vi "AEcollector.vi"() -> ()   [LabVIEW 2009]
panel:
  out "Ch ctrl":bool[](array[boolean])
  out "Channel count":i32
  out "First trigger signal time":timestamp
  out "Boolean 2":bool
  out "# elements in writing queue":i32
  out "Saving data?":bool
  out "Writing loop":bool
  out "Prefilter loop":bool
  out "Collection loop":bool
  out "stateError":bool
  out "stopCollection":bool
  out "# elements in prefiltering queue":i32
  out "Prefiltering loop":i32
  out "Max event amplitude":dbl(knob) scale=0.0..1.0
  out "Data collection loop":i32
  out "data writing loop":i32
  out "Data stream":dynamicdata(graph)
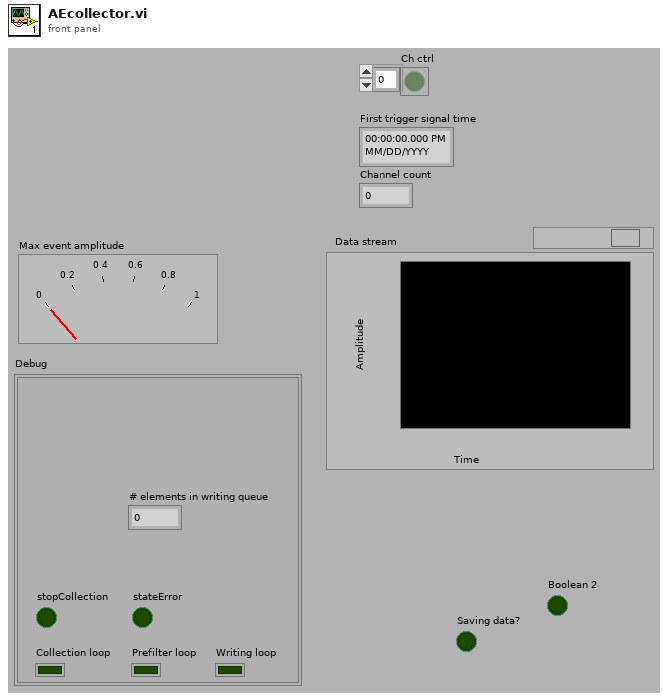
[diagram p1: front panel]
types:
  T1 = enum16{"Read", "Write", "ReadWrite", "BufferedRead", "BufferedReadWrite"}
  T2 = enum16{"open", "replace", "create", "open or create", "replace or create", "replace or create with confirmation"}
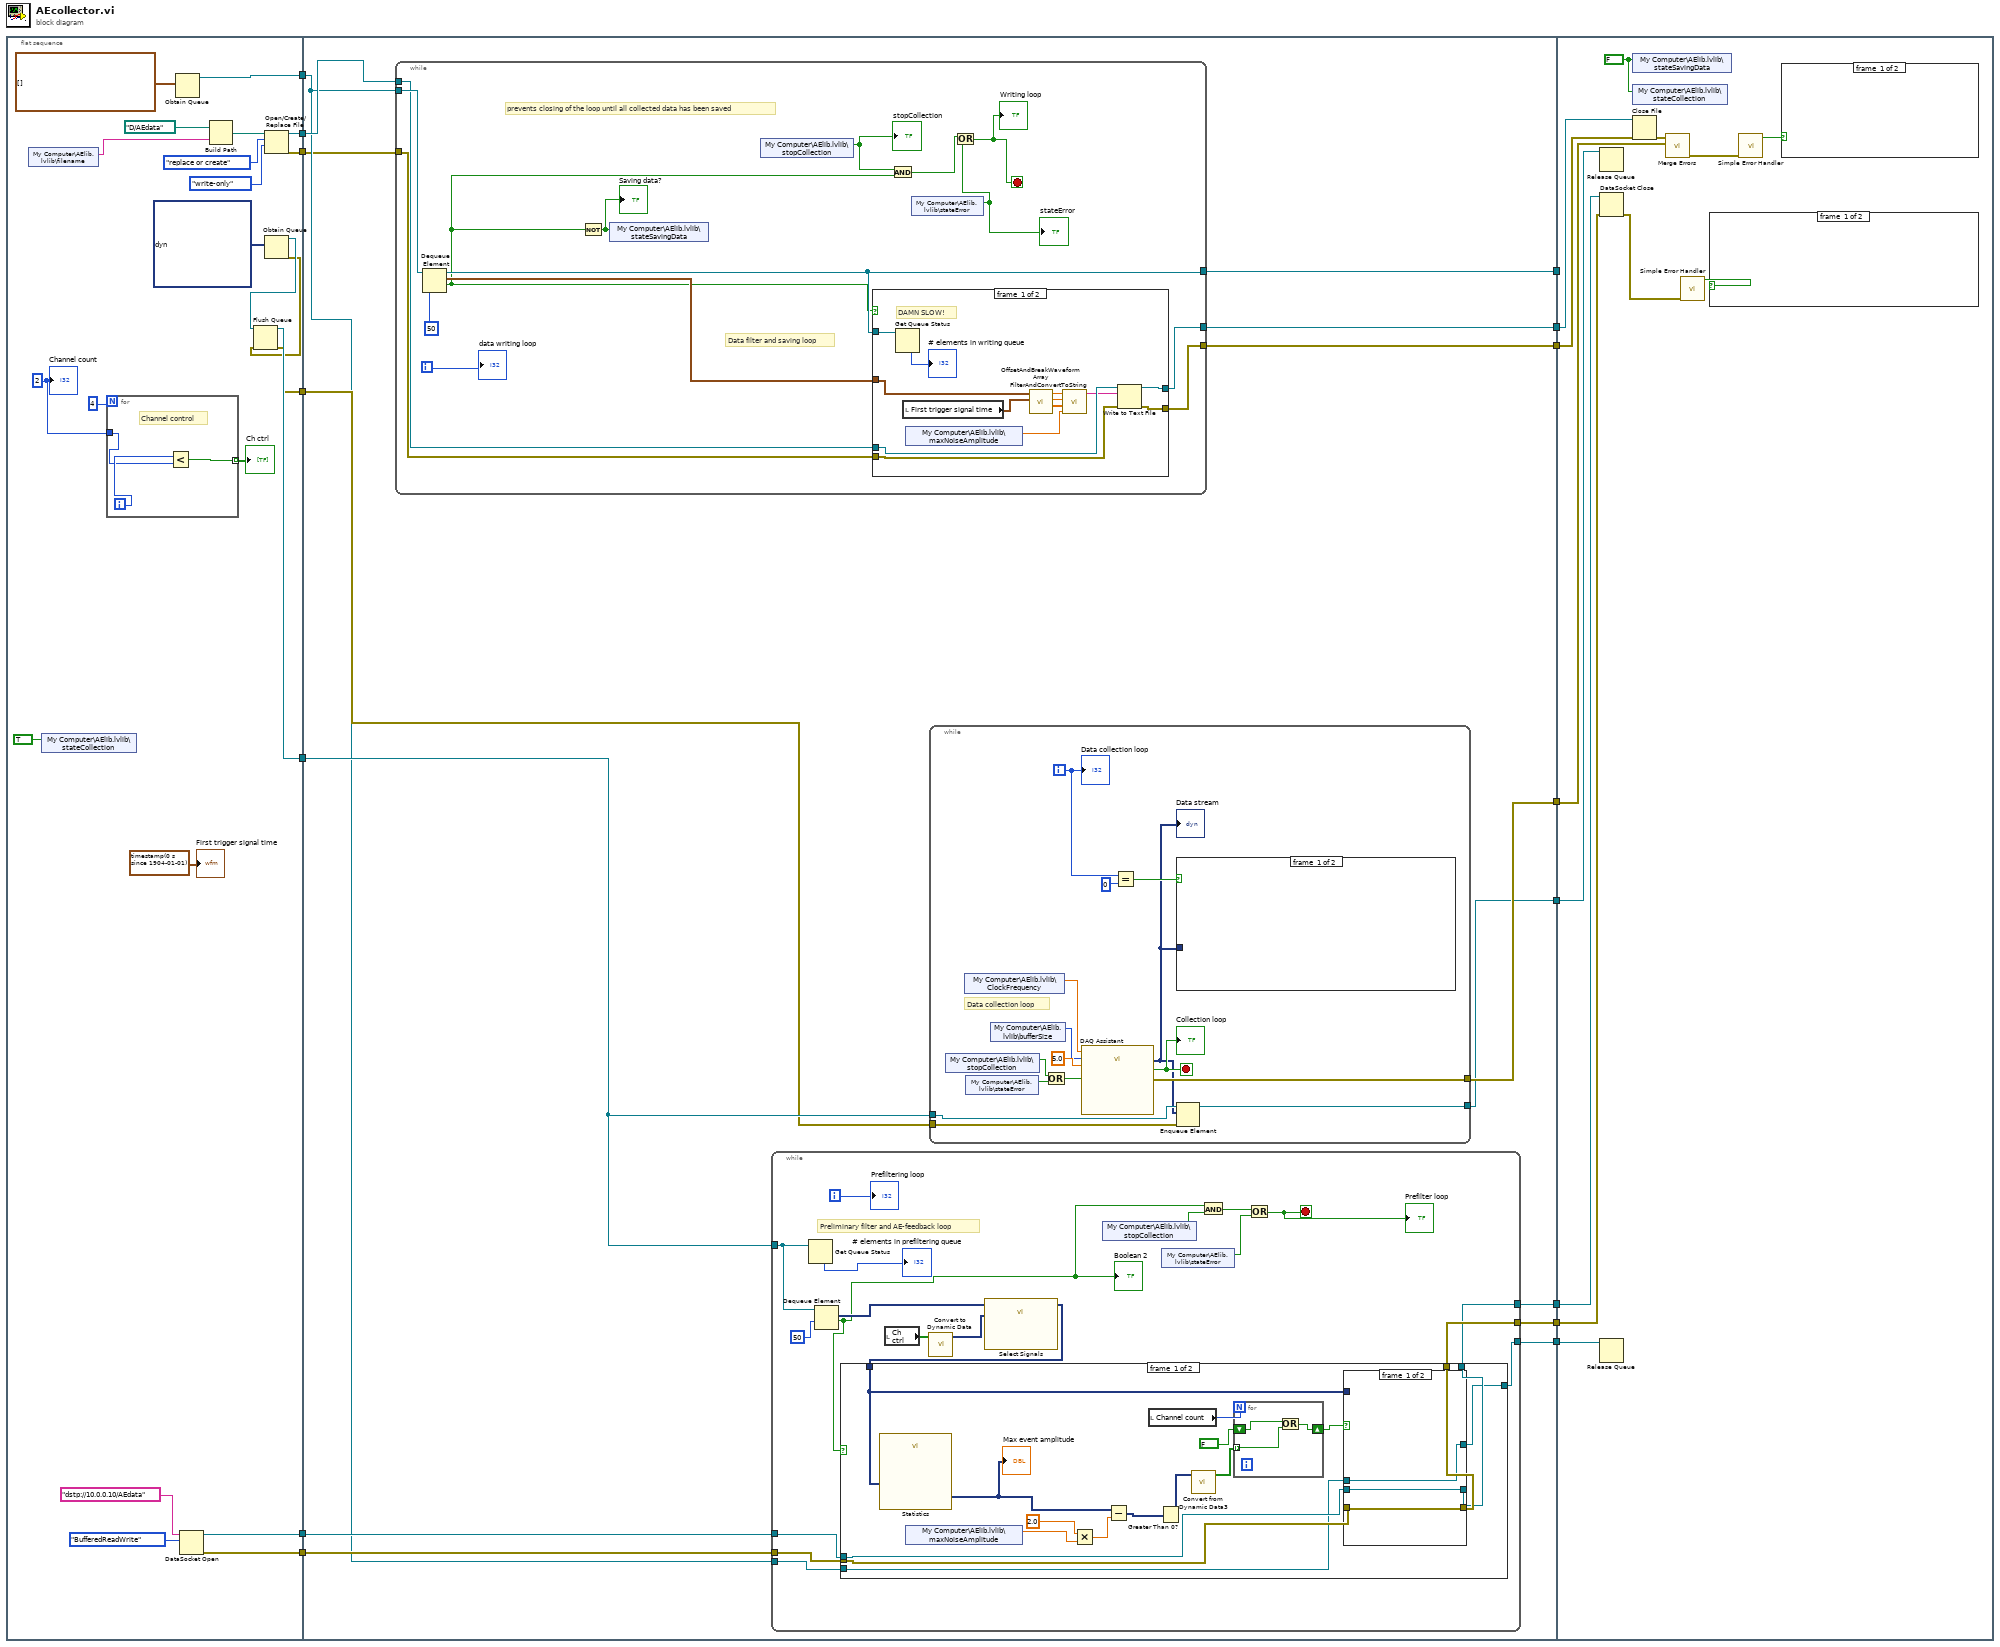
[diagram p0: block diagram]
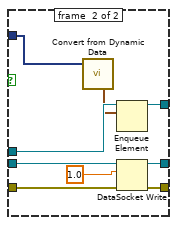
[diagram p2: hidden frame]
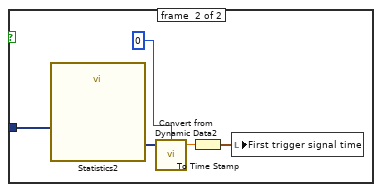
[diagram p5: hidden frame]
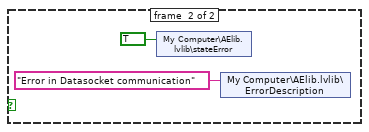
[diagram p6: hidden frame]
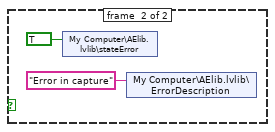
[diagram p7: hidden frame]
diagram:
  n1 = flat-sequence {
    tunnel: [w35] -> w13
    tunnel: [w32] -> w12
    tunnel: [w31] -> w11
    tunnel: [w30] -> w9
    tunnel: [w25] -> w8
    tunnel: [w24] -> w7
    tunnel: [w27] -> w2
    tunnel: [w56] -> w15
    tunnel: [w55] -> w14
    tunnel: w13 -> [w54]
    tunnel: w12 -> [w52]
    tunnel: w11 -> [w53]
    tunnel: [w51] -> w10
    tunnel: w9 -> [w46]
    tunnel: w8 -> [w50]
    tunnel: w7 -> [w49]
    tunnel: [w48] -> w6
    tunnel: [w47] -> w5
    tunnel: [w45] -> w4
    tunnel: [w44] -> w3
    tunnel: w2 -> [w43]
    tunnel: [w42] -> w1
    tunnel: w15 -> [w166]
    tunnel: w14 -> [_]
    tunnel: w10 -> [w172]
    tunnel: w6 -> [w171]
    tunnel: w5 -> [w163]
    tunnel: w4 -> [w170]
    tunnel: w3 -> [w169]
    tunnel: w1 -> [w168]
    frame #0 {
      w19 = 2
      n2 = shared-variable "My Computer\\AElib.lvlib\\filename"() -> (w16:string)  [unwired: 1 in, 1 out]
      n3 = shared-variable "My Computer\\AElib.lvlib\\stateCollection"(TRUE ("stateCollection")) -> ()  [unwired: 1 in, 1 out]
      n4 = for {
        N: 4 -> [_]
        tunnel: w19 -> [w40]
        tunnel: [w39] -> w18 mode=indexing
        i -> [w41]
        # "Channel control"
        n5 = Less?(x=w41, y=w40) -> (x < y?=w39:bool)
      }
      "Ch ctrl" <- w18
      n6 = Obtain Queue(element data type=waveform(dbl)[] []) -> (queue out=w30:refnum<queue>)  [unwired: 4 in, 2 out]
      n7 = DataSocket Open(10:T1."BufferedReadWrite" ("mode"), 11:"dstp://10.0.0.10/AEdata" ("URL")) -> (0:w32:errorcluster, 3:w31:refnum<k13>)  [unwired: 2 in]
      n8 = Build Path(base path=path "D:/AEdata", name or relative path=w16) -> (appended path=w28:path)
      n9 = Open/Create/Replace File(file path (use dialog)=w28, operation (0:open)=T2."replace or create", access (0:read/write)=enum16{"read/write", "read-only", "write-only"}."write-only") -> (refnum out=w35:refnum<file>, error out=w27:errorcluster)  [unwired: 3 in, 1 out]
      n10 = Obtain Queue(element data type=dynamicdata [] ("RMS")) -> (queue out=w26:refnum<queue>, error out=w23:errorcluster)  [unwired: 4 in, 1 out]
      n11 = Flush Queue(queue=w26, error in (no error)=w23) -> (queue out=w25:refnum<queue>, error out=w24:errorcluster)  [unwired: 1 out]
      "First trigger signal time" <- timestamp(0 s since 1904-01-01) ("Time Stamp")
      "Channel count" <- w19
    }
    frame #1 {
      n12 = while {
        tunnel: w54 -> [w115]
        tunnel: w46 -> [w125]
        tunnel: [w117] -> w55
        tunnel: [w114] -> w44
        tunnel: w43 -> [w118]
        tunnel: [w113] -> w42
        i -> [w124]
        stop <- w119 stop-if-true
        # "prevents closing of the loop until all collected data has been saved"
        # "Data filter and saving loop"
        n13 = Dequeue Element(queue=w125, timeout in ms (-1)=50) -> (queue out=w117:refnum<queue>, element=w116:waveform(dbl)[], timed out?=w111:bool)  [unwired: 1 in, 1 out]
        n14 = Not(x=w111) -> (.not. x?=w112:bool)
        "Saving data?" <- w112
        n15 = shared-variable "My Computer\\AElib.lvlib\\stateSavingData"(w112) -> ()  [unwired: 1 in, 1 out]
        n16 = shared-variable "My Computer\\AElib.lvlib\\stopCollection"() -> (w121:bool)  [unwired: 1 in, 1 out]
        "stopCollection" <- w121
        n17 = case shown="False" w111 {
          tunnel: w118 -> [w138 w139]
          tunnel: w117 -> [w133 _]
          tunnel: w116 -> [w132 _]
          tunnel: w115 -> [w137 w140]
          tunnel: [w136 w140] -> w114
          tunnel: [w135 w139] -> w113
          frame #0 {
            # "DAMN SLOW!"
            n18 = Get Queue Status(queue=w133) -> (# elements in queue=→"# elements in writing queue":i32)  [unwired: 2 in, 7 out]
            n19 = local read "First trigger signal time"() -> (w131:timestamp)
            n20 = shared-variable "My Computer\\AElib.lvlib\\maxNoiseAmplitude"() -> (w127:dbl)  [unwired: 1 in, 1 out]
            n21 = call "OffsetAndBreakWaveformArray.vi"("First trigger signal time"=w131, "Array"=w132) -> ("Y"=w128:dbl[][], "dt"=w129:dbl, "t"=w130:dbl)  [unwired: 7 in]
            n22 = call "FilterAndConvertToString.vi"("Max noise amplitude"=w127, "Y"=w128, "dt"=w129, "t"=w130) -> ("String"=w126:string)  [unwired: 7 in]
            n23 = Write to Text File(file (use dialog)=w137, text=w126, error in=w138) -> (refnum out=w136:refnum<file>, error out=w135:errorcluster)  [unwired: 1 in, 1 out]
          }
          frame #1 {
          }
        }
        n24 = And(x=w121, y=w111) -> (x .and. y?=w123:bool)
        n25 = shared-variable "My Computer\\AElib.lvlib\\stateError"() -> (w122:bool)  [unwired: 1 in, 1 out]
        "stateError" <- w122
        n26 = Or(x=w123, y=w122) -> (x .or. y?=w119:bool)
        "Writing loop" <- w119
        "data writing loop" <- w124
      }
      n27 = while {
        tunnel: w53 -> [w73]
        tunnel: w52 -> [w74]
        tunnel: w50 -> [w63]
        tunnel: [w71] -> w48
        tunnel: [w72] -> w47
        tunnel: w46 -> [w70]
        tunnel: [w69] -> w45
        i -> [w68]
        stop <- w65 stop-if-true
        # "Preliminary filter and AE-feedback loop"
        n28 = Get Queue Status(queue=w63) -> (# elements in queue=→"# elements in prefiltering queue":i32)  [unwired: 2 in, 7 out]
        n29 = Dequeue Element(queue=w63, timeout in ms (-1)=50) -> (element=w59:dynamicdata, timed out?=w57:bool)  [unwired: 1 in, 2 out]
        "Boolean 2" <- w57
        n30 = local read "Ch ctrl"() -> (w61:bool[])
        n31 = call "Convert to Dynamic Data"("Array"=w61) -> ("Dynamic Data Type"=w60:dynamicdata)  [unwired: 3 in]
        n32 = call "Select Signals"("Selector Input"=w60, "Signals"=w59) -> ("Signal Out"=w58:dynamicdata)  [unwired: 8 in, 1 out]
        n33 = case shown="False" w57 {
          tunnel: w74 -> [w88 w110]
          tunnel: w73 -> [w87 w108]
          tunnel: [w86 w110] -> w72
          tunnel: [w85 w108] -> w71
          tunnel: w70 -> [w84 w109]
          tunnel: [w83 w109] -> w69
          tunnel: w58 -> [w77 _]
          frame #0 {
            n34 = call "Statistics"("Signals"=w77) -> ("Range"=w76:dynamicdata)  [unwired: 25 in, 1 out]
            "Max event amplitude" <- w76
            n35 = shared-variable "My Computer\\AElib.lvlib\\maxNoiseAmplitude"() -> (w91:dbl)  [unwired: 1 in, 1 out]
            n36 = Multiply(x=2.0, y=w91) -> (x*y=w90:dbl)
            n37 = Subtract(x=w76, y=w90) -> (x-y=w89:dynamicdata)
            n38 = local read "Channel count"() -> (w80:i32)
            n39 = Greater Than 0?(x=w89) -> (x > 0?=w82:dynamicdata)
            n40 = call "Convert from Dynamic Data3"("Dynamic Data Type"=w82) -> ("Array"=w81:bool[])  [unwired: 3 in]
            n41 = for {
              N: w80 -> [_]
              tunnel: w81 -> [w93] mode=indexing
              shift-right: [w95] -> w78
              shift-left: FALSE -> [w94]
              n42 = Or(x=w94, y=w93) -> (x .or. y?=w95:bool)
            }
            n43 = case shown="True" w78 {
              tunnel: w77 -> [_ w99]
              tunnel: w88 -> [w97 w107]
              tunnel: w87 -> [w98 w106]
              tunnel: [w97 w105] -> w86
              tunnel: [w98 w104] -> w85
              tunnel: w84 -> [w96 w103]
              tunnel: [w96 w102] -> w83
              frame #0 {
              }
              frame #1 {
                n44 = call "Convert from Dynamic Data"("Dynamic Data Type"=w99) -> ("Array of Waveform"=w100:waveform(dbl)[])  [unwired: 3 in]
                n45 = Enqueue Element(queue=w103, element=w100) -> (queue out=w102:refnum<queue>)  [unwired: 2 in, 2 out]
                n46 = DataSocket Write(8:w107, 10:1.0 ("x"), 11:w106) -> (0:w105:errorcluster, 3:w104:refnum<k13>)  [unwired: 1 in, 1 out]
              }
            }
          }
          frame #1 {
          }
        }
        n47 = shared-variable "My Computer\\AElib.lvlib\\stopCollection"() -> (w67:bool)  [unwired: 1 in, 1 out]
        n48 = shared-variable "My Computer\\AElib.lvlib\\stateError"() -> (w75:bool)  [unwired: 1 in, 1 out]
        n49 = And(x=w57, y=w67) -> (x .and. y?=w66:bool)
        n50 = Or(x=w66, y=w75) -> (x .or. y?=w65:bool)
        "Prefilter loop" <- w65
        "Prefiltering loop" <- w68
      }
      n51 = while {
        tunnel: [w152] -> w56
        tunnel: w50 -> [w151]
        tunnel: w49 -> [w150]
        tunnel: [w149] -> w51
        i -> [w145]
        stop <- w146 stop-if-true
        # "Data collection loop"
        n52 = shared-variable "My Computer\\AElib.lvlib\\stopCollection"() -> (w155:bool)  [unwired: 1 in, 1 out]
        n53 = shared-variable "My Computer\\AElib.lvlib\\ClockFrequency"() -> (w148:dbl)  [unwired: 1 in, 1 out]
        n54 = shared-variable "My Computer\\AElib.lvlib\\stateError"() -> (w154:bool)  [unwired: 1 in, 1 out]
        n55 = shared-variable "My Computer\\AElib.lvlib\\bufferSize"() -> (w141:i16)  [unwired: 1 in, 1 out]
        n56 = Or(x=w155, y=w154) -> (x .or. y?=w153:bool)
        n57 = call "DAQ Assistant"("rate"=w148, "number of samples"=w141, "timeout (s)"=5.0, "stop (F)"=w153) -> ("data"=w142:dynamicdata, "stopped"=w146:bool, "error out"=w152:errorcluster)  [unwired: 12 in, 1 out]
        "Data stream" <- w142
        "Collection loop" <- w146
        n58 = Equal?(x=w145, y=0) -> (x = y?=w143:bool)
        n59 = case shown="True" w143 {
          tunnel: w142 -> [_ w160]
          frame #0 {
          }
          frame #1 {
            n60 = call "Statistics2"("Signals"=w160) -> ("First Time"=w158:dynamicdata)  [unwired: 25 in, 1 out]
            n61 = call "Convert from Dynamic Data2"("Dynamic Data Type"=w158, "Channel"=0) -> ("Scalar"=w157:dbl)  [unwired: 2 in]
            n62 = To Time Stamp(1:w157) -> (0:w159:timestamp)
            n63 = local write "First trigger signal time"(w159) -> ()
          }
        }
        n64 = Enqueue Element(queue=w151, element=w142, error in (no error)=w150) -> (queue out=w149:refnum<queue>)  [unwired: 1 in, 2 out]
        "Data collection loop" <- w145
      }
    }
    frame #2 {
      w164 = FALSE
      n65 = Release Queue(queue=w172) -> ()  [unwired: 2 in, 3 out]
      n66 = DataSocket Close(8:w163, 11:w171) -> (0:w161:errorcluster)  [unwired: 1 in, 1 out]
      n67 = Release Queue(queue=w170) -> ()  [unwired: 2 in, 3 out]
      n68 = shared-variable "My Computer\\AElib.lvlib\\stateSavingData"(w164) -> ()  [unwired: 1 in, 1 out]
      n69 = shared-variable "My Computer\\AElib.lvlib\\stateCollection"(w164) -> ()  [unwired: 1 in, 1 out]
      n70 = Close File(refnum=w169, error in=w168) -> (error out=w167:errorcluster)  [unwired: 1 out]
      n71 = call <vilib>:"Merge Errors.vi"("error in 2 (no error)"=w166, "error in 1 (no error)"=w167) -> ("error out"=w165:errorcluster)  [unwired: 5 in]
      n72 = call <vilib>:"Simple Error Handler.vi"("error in (no error)"=w161) -> ("error?"=w162:bool)  [unwired: 4 in, 4 out]
      n73 = case shown="True" w162 {
        frame #0 {
        }
        frame #1 {
          n74 = shared-variable "My Computer\\AElib.lvlib\\stateError"(TRUE ("stateError")) -> ()  [unwired: 1 in, 1 out]
          n75 = shared-variable "My Computer\\AElib.lvlib\\ErrorDescription"("Error in Datasocket communication" ("ErrorDescription")) -> ()  [unwired: 1 in, 1 out]
        }
      }
      n76 = call <vilib>:"Simple Error Handler.vi"("error in (no error)"=w165) -> ("error?"=w173:bool)  [unwired: 4 in, 4 out]
      n77 = case shown="True" w173 {
        frame #0 {
        }
        frame #1 {
          n78 = shared-variable "My Computer\\AElib.lvlib\\stateError"(TRUE ("stateError")) -> ()  [unwired: 1 in, 1 out]
          n79 = shared-variable "My Computer\\AElib.lvlib\\ErrorDescription"("Error in capture" ("ErrorDescription")) -> ()  [unwired: 1 in, 1 out]
        }
      }
    }
  }
